vi "Sharp.vi"() -> ()   [LabVIEW 2020]
uses:
  <vilib>/High Genius/HG_WSI_Tookit/Dependencies/Library/Analog In/Analog In.lvclass
  C:/Program Files (x86)/National Instruments/LabVIEW 2020/vi.lib/High Genius/HG_WSI_Tookit/Dependencies/Library/HG_LIB/HG_LIB.lvclass
  <vilib>/Platform/TimedLoop/XDataNode/timing_clust.ctl
  <vilib>/Platform/TimedLoop/XDataNode/nitl_modes.ctl
  <vilib>/Platform/TimedLoop/XDataNode/wakeup.ctl
  <vilib>/platform/TimedLoop/XDataNode/XDataNode.xnode
  <vilib>/High Genius/HG_WSI_Tookit/Dependencies/Library/HG_LIB/HG_LIB.lvclass
  <vilib>/Platform/TimedLoop/XDataNode/XDNodeRunTimeDep.lvlib
panel:
  out "Data":dbl
  out "IR":dbl
  in  "stop":bool
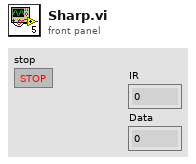
[diagram p1: front panel]
types:
  T1 = enum16{"0", "1", "2", "3", "4", "5", "6", "7", "8", "9", "10", "11", "12", "13", "14", "15", "16", "17", "18", "19", "20", "21", "22", "23", "24", "25"}
  T2 = enum16{"DI", "DO", "AI", "Pulse", "PWM", "ISQ", "ENC", "CAN", "IIC", "IMU"}
  T3 = typedef "XDNodeRunTimeDep.lvlib/timing_clust.ctl" = cluster{"Expected End [f-1]":u64, "Actual End [f-1]":u64, "Finished Late? [f-1]":bool, "Expected End [i-1]":u64, "Actual End [i-1]":u64, "Finished Late? [i-1]":bool, "Expected Start [i]":u64, "Actual Start [i]":u64, "Expected Start [f]":u64, "Actual Start [f]":u64, "Source Name":string, "Structure Name":string, "Period":i64, "Deadline":i64, "Offset":i64, "Start":i64, "Priority":i32, "Timeout":i32, "Mode":T4, "Wakeup Reason":T5, "Error":errorcluster, "Source Type":string, "Secondary Source Type":string, "Global End Time":u64, "Global Start Time":u64, "Frame Duration":u64, "Iteration Duration":u64, "Assigned CPU":i32, "I/O Scan Engine Mode":u32}
  T4 = typedef "XDNodeRunTimeDep.lvlib/nitl_modes.ctl" = enum32{"No Change", "Process missed periods, maintain original phase", "Discard missed periods, maintain original phase", "Process missed periods, ignore original phase", "Discard missed periods, ignore original phase"}
  T5 = typedef "XDNodeRunTimeDep.lvlib/wakeup.ctl" = enum32{"Normal", "Aborted", "Asynchronous wakeup", "Timing source error", "Timed loop error", "Timeout"}
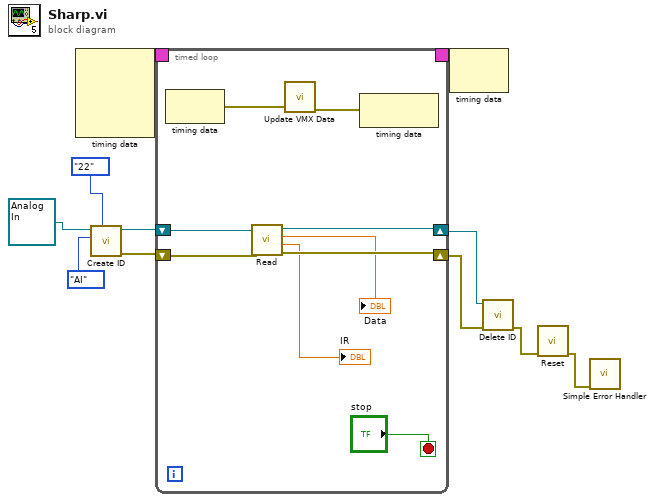
[diagram p0: block diagram]
diagram:
  n1 = node-c288() -> (w11:T3)  [unwired: 4 in]
  n2 = call <vilib>:"Create ID.vi"("NO"=T1."22", "Function"=T2."AI", "HG_LIB in"=refnum<class "Analog In.lvclass"> refnum ("VMX Library.lvlib:Analog In.lvclass")) -> ("error out"=w5:errorcluster, "HG_LIB out"=w6:refnum<class "Analog In.lvclass">)  [unwired: 7 in]
  n3 = timed-loop {
    timing: w11 -> [_]
    timing-out: [_] -> w10
    shift-right: [w15] -> w3
    shift-left: w6 -> [w17]
    shift-right: [w14] -> w4
    shift-left: w5 -> [w16]
    stop <- "stop" stop-if-true
    n4 = node-c288() -> (w19:errorcluster)  [unwired: 1 in]
    n5 = call <vilib>:"Read.vi"("error in (no error)"=w16, "Analog In in"=w17) -> ("error out"=w14:errorcluster, "IR"=→"IR":dbl, "Data"=→"Data":dbl, "Analog In out"=w15:refnum<class "Analog In.lvclass">)  [unwired: 6 in]
    n6 = call <vilib>:"Update VMX Data.vi"("error in (no error)"=w19) -> ("error out"=w18:errorcluster)  [unwired: 10 in]
    n7 = node-c288(w18) -> ()  [unwired: 1 out]
  }
  n8 = node-c288(w10) -> ()  [unwired: 1 out]
  n9 = call <vilib>:"Delete ID.vi"("error in (no error)"=w4, "HG_LIB in"=w3) -> ("error out"=w9:errorcluster)  [unwired: 8 in, 1 out]
  n10 = call <vilib>:"Reset.vi"("error in (no error)"=w9) -> ("error out"=w8:errorcluster)  [unwired: 10 in]
  n11 = call <vilib>:"Simple Error Handler.vi"("error in (no error)"=w8) -> ()  [unwired: 4 in, 5 out]
